vi "MainTypeOO.vi"() -> ()   [LabVIEW 2021]
uses:
  AbstractionMessage/AbstractionMessage.lvclass
  RealWorkActor/RealWorkActor.lvclass
  C:/Users/chrismadlax/Desktop/LVSampleCode/ActorModel/AbstractionActor/AbstractionActor.lvclass
  RealWorkActor/RealWorkActor.lvclass/RealWorkActor.ctl
  UITimeout/UITimeout.lvclass
  ProgramClose/ProgramClose.lvclass
  ActionA/ActionA.lvclass
  ActionB/ActionB.lvclass
  ActionC/ActionC.lvclass
  ProgramInitial/ProgramInitial.lvclass
panel:
  in  "ButtonC":bool
  in  "ButtonB":bool
  in  "ButtonA":bool
  out "NowTime":timestamp
  out "MsgString":string
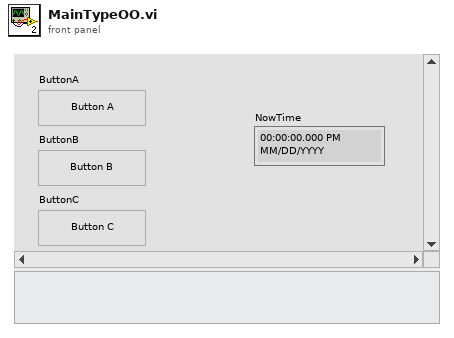
[diagram p1: front panel]
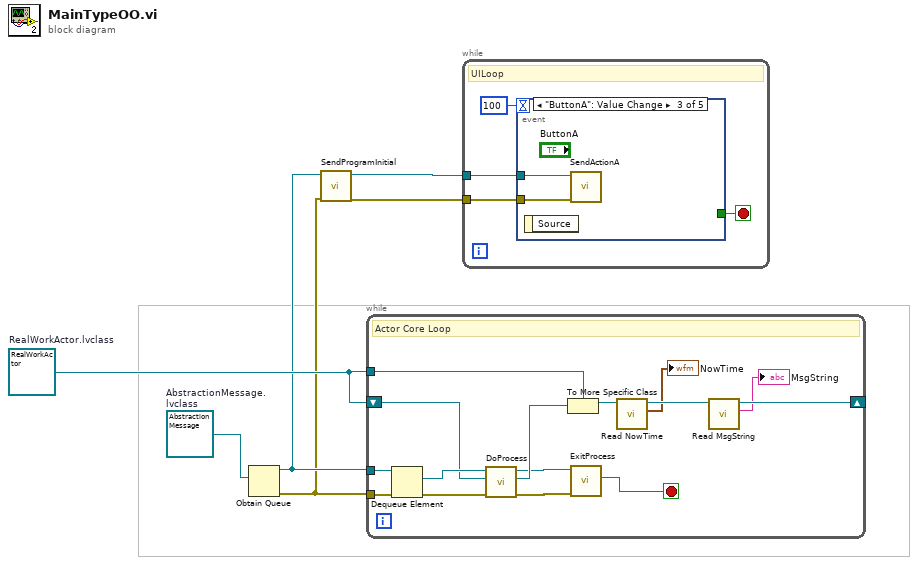
[diagram p0: block diagram]
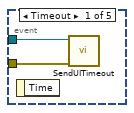
[diagram p2: hidden frame]
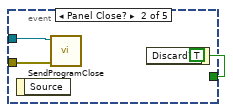
[diagram p3: hidden frame]
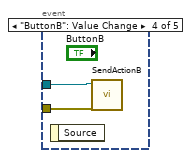
[diagram p4: hidden frame]
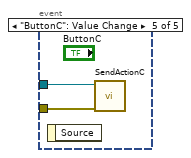
[diagram p5: hidden frame]
diagram:
  w5 = refnum<class "RealWorkActor.lvclass"> refnum  # RealWorkActor.lvclass
  w6 = refnum<class "AbstractionMessage.lvclass"> refnum  # AbstractionMessage.lvclass
  n1 = Obtain Queue(element data type=w6) -> (queue out=w4:refnum<queue>, error out=w3:errorcluster)  [unwired: 4 in, 1 out]
  n2 = call "SendProgramInitial.vi"("error in (no error)"=w3, "Queue in"=w4) -> ("error out"=w2:errorcluster, "Queue out"=w1:refnum<queue>)  [unwired: 8 in]
  n3 = while {
    tunnel: w4 -> [w21]
    tunnel: w3 -> [w20]
    shift-right: [w16] -> _
    shift-left: w5 -> [w17]
    tunnel: w5 -> [w15]
    stop <- w7 stop-if-true
    # "Actor Core Loop"
    n4 = Dequeue Element(queue=w21, error in (no error)=w20) -> (element=w18:refnum<class "AbstractionMessage.lvclass">, error out=w19:errorcluster)  [unwired: 1 in, 2 out]
    n5 = call-dynamic "DoProcess.vi"("error in (no error)"=w19, "AbstractionActor.lvclass"=w17, "AbstractionMessage in"=w18) -> ("error out"=w8:errorcluster, "AbstractionActor.lvclass 2"=w14:refnum<class "AbstractionActor.lvclass">, "AbstractionMessage out"=w9:refnum<class "AbstractionMessage.lvclass">)  [unwired: 6 in]
    n6 = To More Specific Class(target class=w15, reference=w14) -> (specific class reference=w13:refnum<class "RealWorkActor.lvclass">)  [unwired: 1 in, 1 out]
    n7 = call "ExitProcess.vi"("error in (no error)"=w8, "AbstractionMessage in"=w9) -> ("Exit"=w7:bool)  [unwired: 7 in, 2 out]
    n8 = call "Read NowTime.vi"("RealWorkActor in"=w13) -> ("NowTime"=→"NowTime":timestamp, "RealWorkActor out"=w11:refnum<class "RealWorkActor.lvclass">)  [unwired: 8 in, 1 out]
    n9 = call "Read MsgString.vi"("RealWorkActor in"=w11) -> ("MsgString"=→"MsgString":string, "RealWorkActor out"=w16:refnum<class "RealWorkActor.lvclass">)  [unwired: 8 in, 1 out]
  }
  n10 = while {
    tunnel: w1 -> [w24]
    tunnel: w2 -> [w23]
    stop <- w22 stop-if-true
    # "UILoop"
    n11 = event shown="[2] \"ButtonA\": Value Change" {
      selector: _ -> [_ _ _ _ _]
      dyn-events: _ -> [_ _ _ _ _]
      timeout: 100 -> [_ _ _ _ _]
      tunnel: w24 -> [w27 w30 w32 w34 w36]
      tunnel: w23 -> [w26 w29 w31 w33 w35]
      tunnel: [_ w28 _ _ _] -> w22
      event Timeout {
        n12 = event-data() -> ()  [unwired: 1 in, 1 out]
        n13 = call "SendUITimeout.vi"("error in (no error)"=w26, "Queue in"=w27) -> ()  [unwired: 10 in]
      }
      event Panel Close? {
        w28 = TRUE ("Discard?")
        n14 = event-data() -> ()  [unwired: 1 in, 1 out]
        n15 = call "SendProgramClose.vi"("error in (no error)"=w29, "Queue in"=w30) -> ()  [unwired: 10 in]
        n16 = event-data("Discard?"=w28) -> ()  [unwired: 1 in, 1 out]
      }
      event "ButtonA": Value Change {
        n17 = event-data() -> ()  [unwired: 1 in, 1 out]
        n18 = call "SendActionA.vi"("error in (no error)"=w31, "Queue in"=w32) -> ()  [unwired: 10 in]
      }
      event "ButtonB": Value Change {
        n19 = event-data() -> ()  [unwired: 1 in, 1 out]
        n20 = call "SendActionB.vi"("error in (no error)"=w33, "Queue in"=w34) -> ()  [unwired: 10 in]
      }
      event "ButtonC": Value Change {
        n21 = event-data() -> ()  [unwired: 1 in, 1 out]
        n22 = call "SendActionC.vi"("error in (no error)"=w35, "Queue in"=w36) -> ()  [unwired: 10 in]
      }
    }
  }
